vi "point_to_comma.vi"(1 "Lat_A":string) -> (0 "Saída":string)   [LabVIEW 2012]
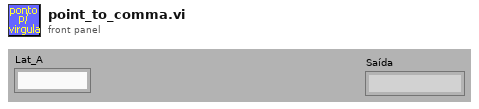
[diagram p1: front panel]
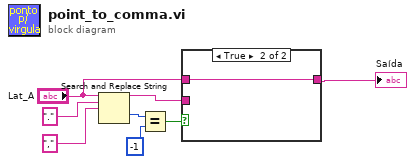
[diagram p0: block diagram]
diagram:
  n1 = Search and Replace String(input string="Lat_A", search string=".", replace string="," ("replace string (\"\")")) -> (result string=w2:string, offset past replacement=w6:i32)  [unwired: 5 in, 2 out]
  n2 = Equal?(x=w6, y=-1) -> (x = y?=w4:bool)
  n3 = case shown="True" w4 {
    tunnel: [w9 w10] -> w1
    tunnel: "Lat_A" -> [_ w10]
    tunnel: w2 -> [w9 _]
    frame False {
    }
    frame True {
    }
  }
  "Saída" <- w1
